vi "Increment Project XML Node Value.vi"(0 "path to XML document":path, 5 "Xpath to Node":string, 11 "error in (no error)":errorcluster) -> (15 "error out":errorcluster)   [LabVIEW 2017, in "CL_G3_VIComponentBuilder.lvlib" / "NI Build Specification_LV.lvclass"]
doc: "Assumes the value of an xml node is a number and increments it."
uses:
  NI Build Specification_LV.lvclass
  <vilib>/xml/Load XML File.vi
  <vilib>/xml/Close Reference(Node).vi
  <vilib>/xml/NI_XML.lvlib
  <resource>/objmgr/DOMUserDefRef.rc
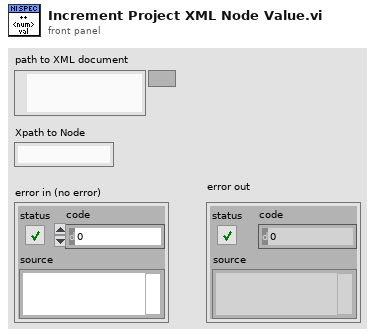
[diagram p1: front panel]
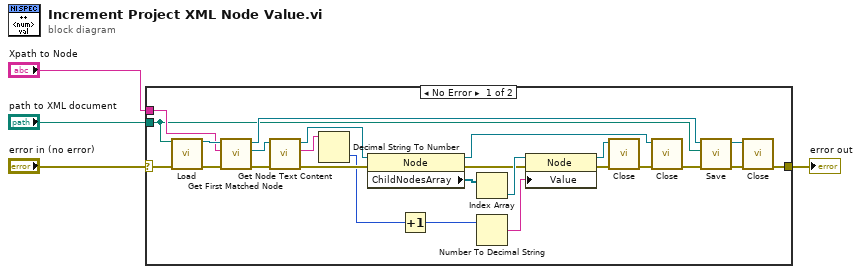
[diagram p0: block diagram]
diagram:
  n1 = case shown="No Error" "error in (no error)" {
    selector: "error in (no error)" -> [w6 w30]
    tunnel: "Xpath to Node" -> [w12 _]
    tunnel: "path to XML document" -> [w11 _]
    tunnel: [w7 w30] -> w2
    frame No Error {
      n2 = call-poly <vilib>:"Load.vi"("path to XML document"=w11, "error in (no error)"=w6) -> ("DOM document out"=w14:refnum<k20>, "error out"=w13:errorcluster)  [unwired: 11 in, 1 out]
      n3 = call <vilib>:"Get First Matched Node.vi"("error in (no error)"=w13, "XPath expression"=w12, "node in"=w14) -> ("error out"=w25:errorcluster, "node result"=w26:refnum<k20>, "node out"=w23:refnum<k20>)  [unwired: 6 in]
      n4 = call <vilib>:"Get Node Text Content.vi"("error in (no error)"=w25, "node in"=w26) -> ("error out"=w21:errorcluster, "node text"=w9:string, "node out"=w24:refnum<k20>)  [unwired: 7 in]
      n5 = Decimal String To Number(string=w9) -> (number=w10:i32)  [unwired: 2 in, 1 out]
      n6 = property class="Node"(reference=w24, error in=w21) -> (reference out=w29:refnum<k20>, error out=w15:errorcluster, "ChildNodesArray"=w20:refnum<k20>[])
      n7 = Increment(x=w10) -> (x+1=w5:i32)
      n8 = Index Array(array=w20) -> (element=w19:refnum<k20>)  [unwired: 1 in]
      n9 = Number To Decimal String(number=w5) -> (decimal integer string=w8:string)  [unwired: 1 in]
      n10 = property class="Node"(reference=w19, error in=w15, "Value"=w8) -> (reference out=w17:refnum<k20>, error out=w18:errorcluster)
      n11 = call-poly <vilib>:"Close.vi"("error in (no error)"=w18, "node"=w17) -> ("error out"=w16:errorcluster)  [unwired: 7 out]
      n12 = call-poly <vilib>:"Close.vi"("error in (no error)"=w16, "node"=w29) -> ("error out"=w22:errorcluster)  [unwired: 7 in]
      n13 = call <vilib>:"Save.vi"("error in (no error)"=w22, "XML file path"=w11, "DOM document in"=w23) -> ("error out"=w27:errorcluster, "DOM document out"=w28:refnum<k20>)  [unwired: 6 in, 1 out]
      n14 = call-poly <vilib>:"Close.vi"("error in (no error)"=w27, "node"=w28) -> ("error out"=w7:errorcluster)  [unwired: 7 in]
    }
    frame Error {
    }
  }
  "error out" <- w2
